vi "ensure connection to slaves.vi"(7 "delay":u32=100, 8 "error in":errorcluster, 9 "Timeout (ms)":i32=-1, 10 "Slave Info List":T1(array[cluster]), 11 "profibus reference":T2) -> (0 "error out":errorcluster, 3 "profibus reference out":T2)   [LabVIEW 2013, in "dynamic profibus.lvlib"]
uses:
  dynamic profibus.lvlib
  fpga reference.ctl
  profibus master action.ctl
  profibus master transmit header.ctl
  <vilib>/rvi/interface/common/niFpgaWaitOnOcc.vi
  <vilib>/Utility/error.llb/Error Cluster From Error Code.vi
  <vilib>/rvi/errors/niLvFpgaAdjustHostInterfaceError.vi
  <vilib>/rvi/interface/nirviMethod/nirviMethod.xnode
  <vilib>/rvi/errors/niLvFpgaMergeErrorWithErrorCode.vi
  <vilib>/FPGAPlugInAG/Dynamic/niLvFpga_WriteFifo_Dynamic.vi
  <vilib>/FPGAPlugInAG/Dynamic/niLvFpga_ReadFifo_Dynamic.vi
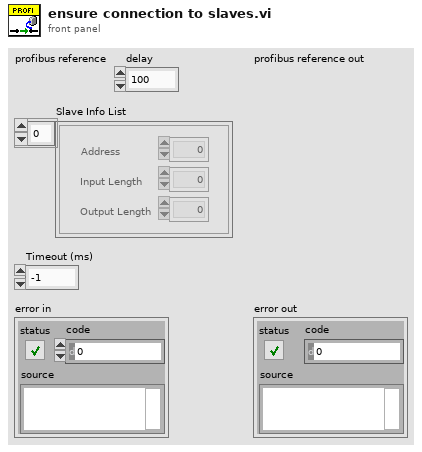
[diagram p1: front panel]
types:
  T1 = cluster{"Address":i8, "Input Length":u8, "Output Length":u8}[]
  T2 = typedef "dynamic profibus.lvlib/fpga reference.ctl" = refnum<k20>
  T3 = typedef "dynamic profibus.lvlib/profibus master action.ctl" = enum8{"initialize", "uninitialize", "stop", "get input", "get input size", "set output", "get output size", "get diagnostic", "transfer data", "transfer diagnostics", "read many inputs"}
  T4 = typedef "dynamic profibus.lvlib/profibus master transmit header.ctl" = enum8{"Error", "Input", "Diagnostic", "input size", "output size", "many inputs"}
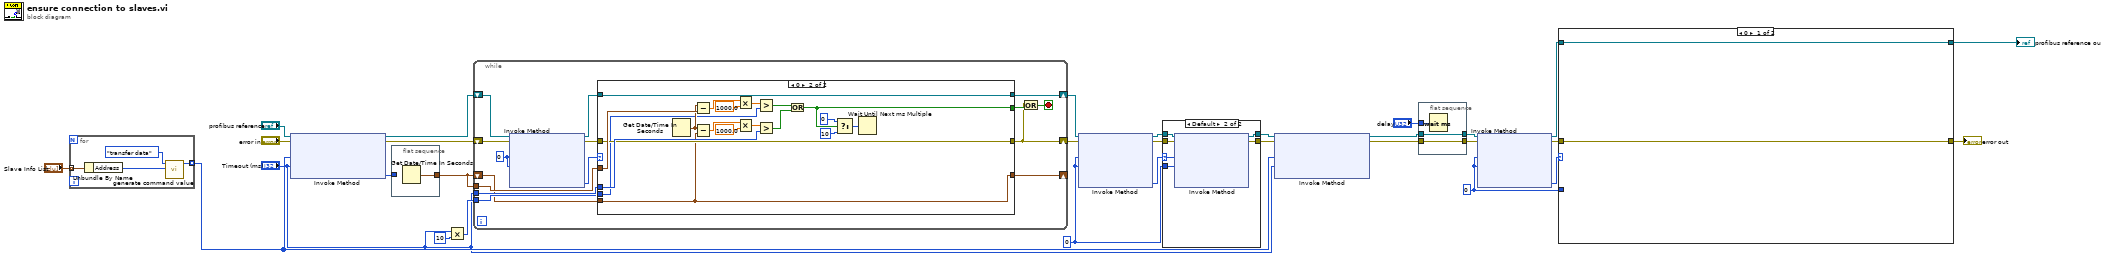
[diagram p0: block diagram]
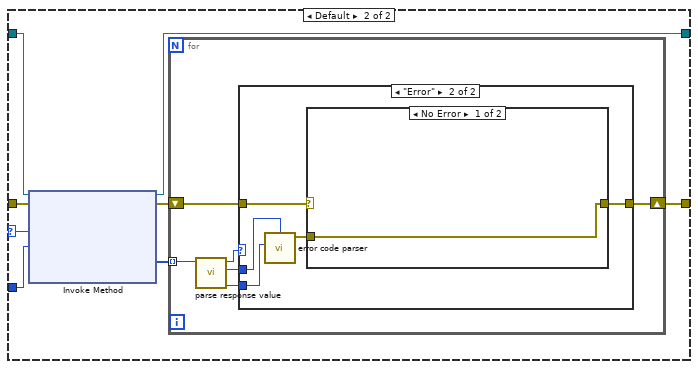
[diagram p2: hidden frame]
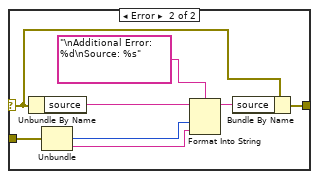
[diagram p4: hidden frame]
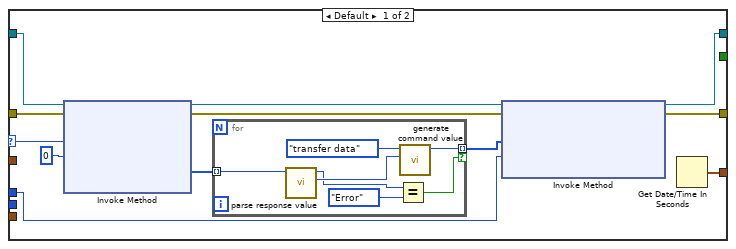
[diagram p6: hidden frame]
diagram:
  w8 = 0 ("Timeout (ms)")
  w16 = 0 ("Timeout (ms)")
  n1 = for {
    tunnel: "Slave Info List" -> [w34] mode=indexing
    tunnel: [w31] -> w13 mode=indexing
    n2 = Unbundle By Name(w34) -> ("Address"=w32:i8)
    n3 = call "generate command value.vi"("device"=w32, "action"=profibus_master_action."transfer data") -> ("Element"=w31:u32)  [unwired: 9 in]
  }
  n4 = xnode "Invoke Method"("FPGA VI Reference In"="profibus reference", "error in"="error in", "Data"=w13, "Timeout (ms)"="Timeout (ms)") -> ("FPGA VI Reference Out"=w27:T2, "error out"=w26:errorcluster, "Empty Elements Remaining"=w25:u32)
  n5 = flat-sequence {
    tunnel: w25 -> [_]
    tunnel: [w35] -> w22
    frame #0 {
      n6 = Get Date/Time In Seconds() -> (seconds since 1Jan1904=w35:timestamp)
    }
  }
  n7 = Multiply(x="Timeout (ms)", y=10) -> (x*y=w23:i32)
  n8 = while {
    shift-right: [w46] -> w19
    shift-left: w27 -> [w50]
    tunnel: w22 -> [w44]
    tunnel: "Timeout (ms)" -> [w43]
    shift-right: [w39] -> w18
    shift-left: w26 -> [w49]
    tunnel: w23 -> [w38]
    shift-right: [w36] -> _
    shift-left: w22 -> [w37]
    stop <- w40 stop-if-true
    w48 = u32 0 ("Number of Elements")
    n9 = xnode "Invoke Method"("FPGA VI Reference In"=w50, "error in"=w49, "Number of Elements"=w48, "Timeout (ms)"=w48) -> ("FPGA VI Reference Out"=w45:T2, "error out"=w41:errorcluster, "Elements Remaining"=w47:u32)  [unwired: 1 out]
    n10 = case shown="0" w47 {
      selector: w47 -> [w59 _]
      tunnel: [w57 w88] -> w46
      tunnel: w45 -> [w62 w88]
      tunnel: w44 -> [_ w87]
      tunnel: w43 -> [w51 w84]
      tunnel: [_ w78] -> w42
      tunnel: w41 -> [w61 w79]
      tunnel: [w56 w79] -> w39
      tunnel: w38 -> [_ w74]
      tunnel: w37 -> [_ w72]
      tunnel: [w60 w72] -> w36
      frame Default {
        n11 = xnode "Invoke Method"("FPGA VI Reference In"=w62, "error in"=w61, "Number of Elements"=w59, "Timeout (ms)"=0) -> ("FPGA VI Reference Out"=w55:T2, "error out"=w54:errorcluster, "Data"=w53:u32[])  [unwired: 1 out]
        n12 = for {
          tunnel: w53 -> [w69] mode=indexing
          tunnel: [w66] -> w52 mode=indexing if=w63
          n13 = call "parse response value.vi"("Element"=w69) -> ("device"=w67:u8, "header"=w65:T4)  [unwired: 7 in, 2 out]
          n14 = Equal?(x=w65, y=profibus_master_transmit_header."Error") -> (x = y?=w63:bool)
          n15 = call "generate command value.vi"("device"=w67, "action"=profibus_master_action."transfer data") -> ("Element"=w66:u32)  [unwired: 9 in]
        }
        n16 = xnode "Invoke Method"("FPGA VI Reference In"=w55, "error in"=w54, "Data"=w52, "Timeout (ms)"=w51) -> ("FPGA VI Reference Out"=w57:T2, "error out"=w56:errorcluster)  [unwired: 1 out]
        n17 = Get Date/Time In Seconds() -> (seconds since 1Jan1904=w60:timestamp)
      }
      frame 0 {
        n18 = Get Date/Time In Seconds() -> (seconds since 1Jan1904=w75:timestamp)
        n19 = Subtract(x=w75, y=w87) -> (x-y=w86:dbl)
        n20 = Subtract(x=w75, y=w72) -> (x-y=w76:dbl)
        n21 = Multiply(x=w86, y=1000.0) -> (x*y=w71:dbl)
        n22 = Multiply(x=w76, y=1000.0) -> (x*y=w70:dbl)
        n23 = Greater?(x=w71, y=w74) -> (0:w73:bool)
        n24 = Greater?(x=w70, y=w84) -> (0:w83:bool)
        n25 = Or(x=w73, y=w83) -> (x .or. y?=w78:bool)
        n26 = Select(t=u32 0 ("millisecond multiple"), s=w78, f=u32 10 ("millisecond multiple")) -> (s? t:f=w82:u32)
        n27 = Wait Until Next ms Multiple(millisecond multiple=w82) -> ()  [unwired: 1 out]
      }
    }
    n28 = Or(x=w39, y=w42) -> (x .or. y?=w40:bool)
  }
  n29 = xnode "Invoke Method"("FPGA VI Reference In"=w19, "error in"=w18, "Number of Elements"=w16, "Timeout (ms)"=w16) -> ("FPGA VI Reference Out"=w21:T2, "error out"=w20:errorcluster, "Elements Remaining"=w17:u32)  [unwired: 1 out]
  n30 = case shown="Default" w17 {
    selector: w17 -> [_ w92]
    tunnel: w21 -> [w90 w96]
    tunnel: w20 -> [w89 w95]
    tunnel: [w90 w94] -> w15
    tunnel: [w89 w93] -> w14
    tunnel: w16 -> [_ w91]
    frame 0 {
    }
    frame Default {
      n31 = xnode "Invoke Method"("FPGA VI Reference In"=w96, "error in"=w95, "Number of Elements"=w92, "Timeout (ms)"=w91) -> ("FPGA VI Reference Out"=w94:T2, "error out"=w93:errorcluster)  [unwired: 2 out]
    }
  }
  n32 = xnode "Invoke Method"("FPGA VI Reference In"=w15, "error in"=w14, "Data"=w13, "Timeout (ms)"="Timeout (ms)") -> ("FPGA VI Reference Out"=w10:T2, "error out"=w11:errorcluster)  [unwired: 1 out]
  n33 = flat-sequence {
    tunnel: [w99] -> w3
    tunnel: w11 -> [w99]
    tunnel: w10 -> [w98]
    tunnel: [w98] -> w4
    tunnel: "delay" -> [w97]
    frame #0 {
      n34 = Wait (ms)(milliseconds to wait=w97) -> ()  [unwired: 1 out]
    }
  }
  n35 = xnode "Invoke Method"("FPGA VI Reference In"=w4, "error in"=w3, "Number of Elements"=w8, "Timeout (ms)"=w8) -> ("FPGA VI Reference Out"=w5:T2, "error out"=w6:errorcluster, "Elements Remaining"=w7:u32)  [unwired: 1 out]
  n36 = case shown="0" w7 {
    selector: w7 -> [_ w107]
    tunnel: w5 -> [w101 w109]
    tunnel: w6 -> [w100 w108]
    tunnel: [w101 w102] -> w2
    tunnel: [w100 w103] -> w1
    tunnel: w8 -> [_ w106]
    frame 0 {
    }
    frame Default {
      n37 = xnode "Invoke Method"("FPGA VI Reference In"=w109, "error in"=w108, "Number of Elements"=w107, "Timeout (ms)"=w106) -> ("FPGA VI Reference Out"=w102:T2, "error out"=w105:errorcluster, "Data"=w104:u32[])  [unwired: 1 out]
      n38 = for {
        shift-right: [w112] -> w103
        shift-left: w105 -> [w115]
        tunnel: w104 -> [w114] mode=indexing
        n39 = call "parse response value.vi"("Element"=w114) -> ("data"=w111:u8, "device"=w110:u8, "header"=w113:T4)  [unwired: 7 in, 1 out]
        n40 = case shown="\"Error\"" w113 {
          tunnel: w115 -> [w116 w120]
          tunnel: [w116 w119] -> w112
          tunnel: w111 -> [_ w121]
          tunnel: w110 -> [_ w117]
          frame Default {
          }
          frame "Error" {
            n41 = call "error code parser.vi"("device"=w117, "Status"=w121) -> ("Error out"=w118:errorcluster)  [unwired: 7 in]
            n42 = case shown="No Error" w120 {
              selector: w120 -> [_ w130]
              tunnel: [w122 w129] -> w119
              tunnel: w118 -> [w122 w128]
              frame No Error {
              }
              frame Error {
                n43 = Unbundle By Name(w130) -> ("source"=w127:string)
                n44 = Unbundle(w128) -> ("code"=w124:i32, "source"=w123:string)  [unwired: 1 out]
                n45 = Format Into String(format string="\nAdditional Error: %d\nSource: %s", initial string=w127, w124, w123) -> (resulting string=w126:string)  [unwired: 1 in, 1 out]
                n46 = Bundle By Name(cluster=w130, "source"=w126) -> (w129:errorcluster)
              }
            }
          }
        }
      }
    }
  }
  "error out" <- w1
  "profibus reference out" <- w2
